vi "TwoBallAutoMoat.vi"   [LabVIEW 2015]
uses:
  <vilib>/Rock Robotics/WPI/DriverStation/WPI_DriverStationRobotMode2.ctl
  Utilities/MotorPositionGlobals.vi
  Utilities/AutoVars.vi
  TwoBallAutoGlobals.vi
  navx-mxp/labview/navX Library v2/navX Library v2.lvlib
types:
  T1 = enum16{"WaitForInput", "StartIntake", "LowerArm", "IntakeBall", "TurnAndZeroEnc", "DriveForward", "RecordGyro", "TargetAndLoad", "Shoot", "TurnBack", "BackUpAndIntake", "IntakeBall2", "DriveForward2", "TargetAndLoad2", "Shoot2", "End"}
  T2 = typedef "WPI_DriverStationRobotMode2.ctl" = enum16{"Autonomous Disabled", "Autonomous Enabled", "Teleop Disabled", "Teleop Enabled", "Disconnected", "Finish", "Test Disabled", "Test Enabled", "Emergency Stopped"}
  T3 = typedef "WPI_MotorControlDeviceRef.ctl" = cluster{"DeviceStatus":errorcluster, "Type":T4, "PWM":cluster{"PWM Channel":T5, "DeadBand":T6}, "CAN":cluster{"Device Number":u8, "Control Mode":T7, "Semaphore":T8, "Max Vout":dbl, "TalonSRX Control Mode":T9}, "Invert":bool}
  T4 = typedef "WPI_MotorControlType.ctl" = enum16{"PWM", "CAN", "CANTalonSRX"}
  T5 = typedef "FPGA_DIOPWMChannel.ctl" = enum8{"PWM 0", "PWM 1", "PWM 2", "PWM 3", "PWM 4", "PWM 5", "PWM 6", "PWM 7", "PWM 8", "PWM 9", "PWM MXP 0", "PWM MXP 1", "PWM MXP 2", "PWM MXP 3", "PWM MXP 4", "PWM MXP 5", "PWM MXP 6", "PWM MXP 7", "PWM MXP 8", "PWM MXP 9", "Invalid"}
  T6 = typedef "WPI_PWMDeadband.ctl" = cluster{"Name":string, "maxPositivePwm":i32, "minPositivePwm":i32, "centerPwm":i32, "maxNegativePwm":i32, "minNegativePwm":i32, "angularRange":u16}
  T7 = typedef "WPI_CANJaguar_ControlMode.ctl" = enum8{"Percent VBus", "Current", "Speed", "Position", "Voltage"}
  T8 = typedef "Semaphore RefNum" = refnum<k1>
  T9 = typedef "WPI_CANTalonSRX_APIControlMode.ctl" = enum8{"Percent VBus", "Speed", "Position", "Slave", "Unchanged / Invalid", "Voltage Compensation", "Current", "Motion Profile"}
  T10 = typedef "navX Library v2.lvlib/Z900_navX_DeviceTypeDef.ctl" = cluster{"Interface":cluster{"Protocol":T11, "Update Rate (4Hz-60Hz)":u8, "navX Open TypeDef":variant}, "Notify Packet":refnum<notifier>, "Loop VI Refnum":refnum<vi>, "Ready to Close Occurrence Refnum":refnum<k4>}
  T11 = typedef "navX Library v2.lvlib/Z900_navX_ProtocolTypeDef.ctl" = enum16{"SERIAL", "I2C", "SPI"}
  T12 = cluster{"Yaw":dbl, "Roll":dbl, "Pitch":dbl, "Heading":dbl, "Fused Heading":dbl}
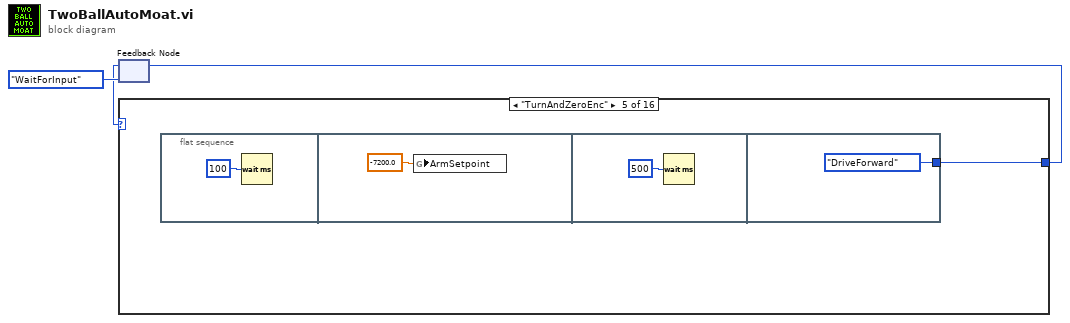
[diagram p0: block diagram]
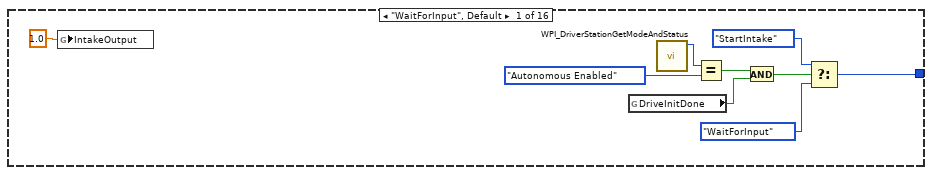
[diagram p2: hidden frame]
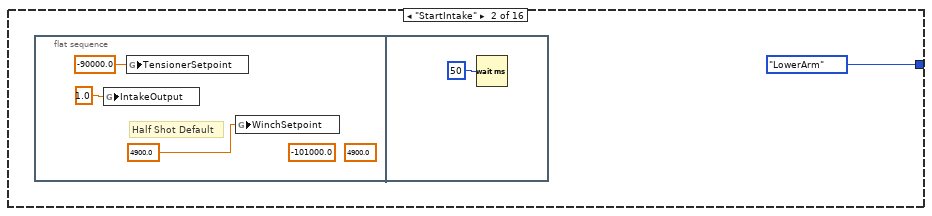
[diagram p3: hidden frame]
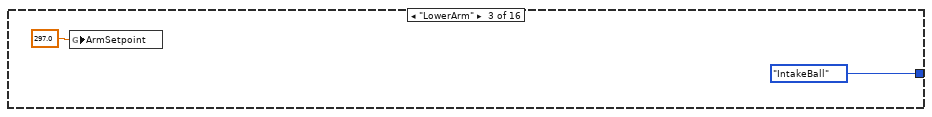
[diagram p4: hidden frame]
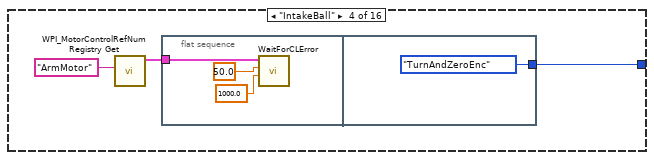
[diagram p5: hidden frame]
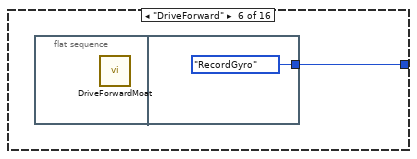
[diagram p6: hidden frame]
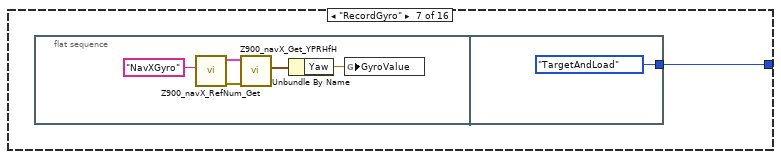
[diagram p7: hidden frame]
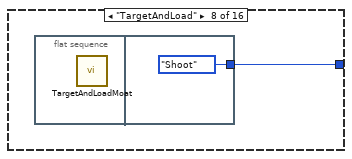
[diagram p8: hidden frame]
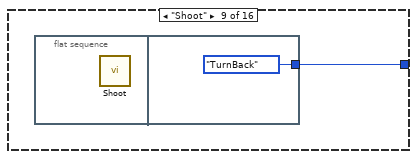
[diagram p9: hidden frame]
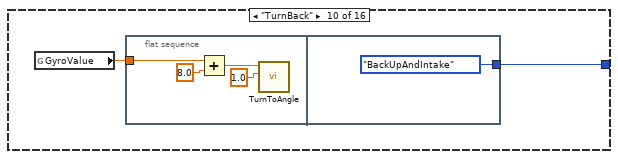
[diagram p10: hidden frame]
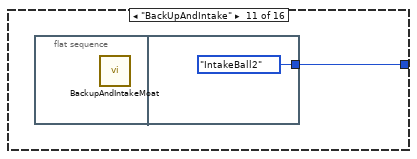
[diagram p11: hidden frame]
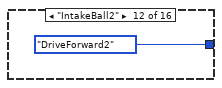
[diagram p12: hidden frame]
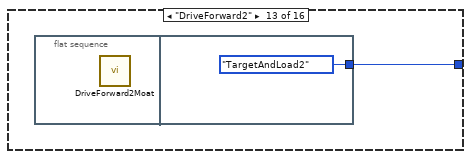
[diagram p13: hidden frame]
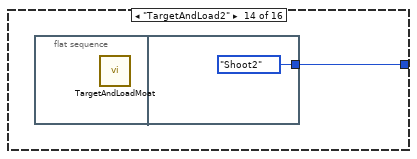
[diagram p14: hidden frame]
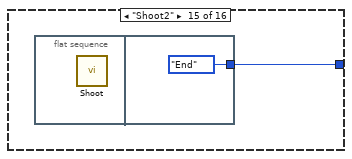
[diagram p15: hidden frame]
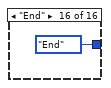
[diagram p16: hidden frame]
diagram:
  n1 = feedback #1(T1."WaitForInput" ("Enum")) -> (w1:T1)
  n2 = case shown="\"TurnAndZeroEnc\"" w1 {
    tunnel: [w5 T1."LowerArm" ("Enum") T1."IntakeBall" ("Enum") w22 w27 w32 w34 w41 w43 w45 w52 T1."DriveForward2" ("Enum") w55 w57 w59 T1."End" ("Enum")] -> w3
    frame "WaitForInput", Default {
      n3 = global write "MotorPositionGlobals.vi" "IntakeOutput"(1.0 ("IntakeOutput")) -> ()
      n4 = global read "AutoVars.vi" "DriveInitDone"() -> (w9:bool)
      n5 = call <vilib>:"WPI_DriverStationGetModeAndStatus.vi"() -> ("Robot Mode"=w12:T2)  [unwired: 10 in, 1 out]
      n6 = Equal?(x=w12, y=WPI_DriverStationRobotMode2."Autonomous Enabled" ("Robot Mode")) -> (x = y?=w10:bool)
      n7 = And(x=w10, y=w9) -> (x .and. y?=w8:bool)
      n8 = Select(t=T1."StartIntake" ("Enum"), s=w8, f=T1."WaitForInput" ("Enum")) -> (s? t:f=w5:T1)
    }
    frame "StartIntake" {
      n9 = flat-sequence {
        frame #0 {
          (unwired) 4900.0 ("WinchPosition")
          (unwired) -101000.0 ("TensionerSetpoint")
          # "Half Shot Default"
          n10 = global write "MotorPositionGlobals.vi" "IntakeOutput"(1.0 ("IntakeOutput")) -> ()
          n11 = global write "MotorPositionGlobals.vi" "TensionerSetpoint"(-90000.0 ("TensionerSetpoint")) -> ()
          n12 = global write "MotorPositionGlobals.vi" "WinchSetpoint"(4900.0 ("WinchPosition")) -> ()
        }
        frame #1 {
          n13 = Wait (ms)(milliseconds to wait=u32 50) -> ()  [unwired: 1 out]
        }
      }
    }
    frame "LowerArm" {
      n14 = global write "MotorPositionGlobals.vi" "ArmSetpoint"(297.0 ("ArmSetpoint")) -> ()
    }
    frame "IntakeBall" {
      n15 = call <vilib>:"WPI_MotorControlRefNum Registry Get.vi"("refnum name"="ArmMotor") -> ("MotorControlDevRef"=w20:T3)  [unwired: 9 in, 1 out]
      n16 = flat-sequence {
        tunnel: w20 -> [w25]
        tunnel: [T1."TurnAndZeroEnc" ("Enum")] -> w22
        frame #0 {
          n17 = call "WaitForCLError.vi"("Timeout (ms)"=1000.0, "AllowedError"=50.0, "CAN Talon SRX Ref"=w25) -> ()  [unwired: 8 in, 1 out]
        }
        frame #1 {
        }
      }
    }
    frame "TurnAndZeroEnc" {
      n18 = flat-sequence {
        tunnel: [T1."DriveForward" ("Enum")] -> w27
        frame #0 {
          n19 = Wait (ms)(milliseconds to wait=u32 100) -> ()  [unwired: 1 out]
        }
        frame #1 {
          n20 = global write "MotorPositionGlobals.vi" "ArmSetpoint"(-7200.0 ("ArmSetpoint")) -> ()
        }
        frame #2 {
          n21 = Wait (ms)(milliseconds to wait=u32 500) -> ()  [unwired: 1 out]
        }
        frame #3 {
        }
      }
    }
    frame "DriveForward" {
      n22 = flat-sequence {
        tunnel: [T1."RecordGyro" ("Enum")] -> w32
        frame #0 {
          n23 = call "DriveForwardMoat.vi"() -> ()  [unwired: 12 in]
        }
        frame #1 {
        }
      }
    }
    frame "RecordGyro" {
      n24 = flat-sequence {
        tunnel: [T1."TargetAndLoad" ("Enum")] -> w34
        frame #0 {
          n25 = call "Z900_navX_RefNum_Get.vi"("refnum name"="NavXGyro") -> ("error out"=w38:errorcluster, "navX Device"=w39:T10)  [unwired: 9 in]
          n26 = call "Z900_navX_Get_YPRHfH.vi"("error in (no error)"=w38, "navX Device"=w39) -> ("YRPHfH"=w36:T12)  [unwired: 6 in, 3 out]
          n27 = Unbundle By Name(w36) -> ("Yaw"=w35:dbl)
          n28 = global write "TwoBallAutoGlobals.vi" "GyroValue"(w35) -> ()
        }
        frame #1 {
        }
      }
    }
    frame "TargetAndLoad" {
      n29 = flat-sequence {
        tunnel: [T1."Shoot" ("Enum")] -> w41
        frame #0 {
          n30 = call "TargetAndLoadMoat.vi"() -> ()  [unwired: 1 in]
        }
        frame #1 {
        }
      }
    }
    frame "Shoot" {
      n31 = flat-sequence {
        tunnel: [T1."TurnBack" ("Enum")] -> w43
        frame #0 {
          n32 = call "Shoot.vi"() -> ()  [unwired: 12 in]
        }
        frame #1 {
        }
      }
    }
    frame "TurnBack" {
      n33 = global read "TwoBallAutoGlobals.vi" "GyroValue"() -> (w46:dbl)
      n34 = flat-sequence {
        tunnel: w46 -> [w49]
        tunnel: [T1."BackUpAndIntake" ("Enum")] -> w45
        frame #0 {
          n35 = Add(x=w49, y=8.0) -> (x+y=w48:dbl)
          n36 = call "TurnToAngle.vi"("AllowedDeviation"=1.0, "GyroValue"=w48) -> ()  [unwired: 10 in]
        }
        frame #1 {
        }
      }
    }
    frame "BackUpAndIntake" {
      n37 = flat-sequence {
        tunnel: [T1."IntakeBall2" ("Enum")] -> w52
        frame #0 {
          n38 = call "BackupAndIntakeMoat.vi"() -> ()  [unwired: 2 in]
        }
        frame #1 {
        }
      }
    }
    frame "IntakeBall2" {
    }
    frame "DriveForward2" {
      n39 = flat-sequence {
        tunnel: [T1."TargetAndLoad2" ("Enum")] -> w55
        frame #0 {
          n40 = call "DriveForward2Moat.vi"() -> ()  [unwired: 2 in]
        }
        frame #1 {
        }
      }
    }
    frame "TargetAndLoad2" {
      n41 = flat-sequence {
        tunnel: [T1."Shoot2" ("Enum")] -> w57
        frame #0 {
          n42 = call "TargetAndLoadMoat.vi"() -> ()  [unwired: 1 in]
        }
        frame #1 {
        }
      }
    }
    frame "Shoot2" {
      n43 = flat-sequence {
        tunnel: [T1."End" ("Enum")] -> w59
        frame #0 {
          n44 = call "Shoot.vi"() -> ()  [unwired: 12 in]
        }
        frame #1 {
        }
      }
    }
    frame "End" {
    }
  }
  n45 = feedback-in #1(w3) -> ()
